vi "Split Host Port.vi"(10 "Address":string) -> (1 "Port":i32, 2 "Hostname":string)   [LabVIEW 2024, in "Sift Client.lvlib" / "Sift Client.lvclass"]
uses:
  Sift Client.lvclass
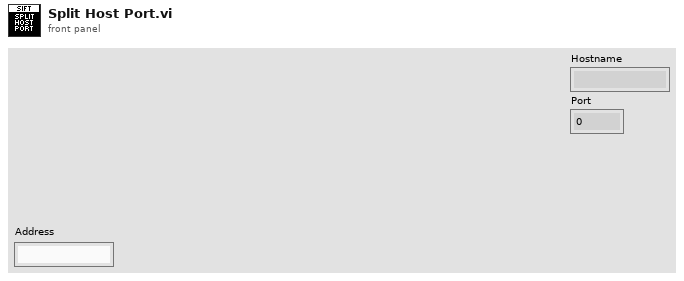
[diagram p1: front panel]
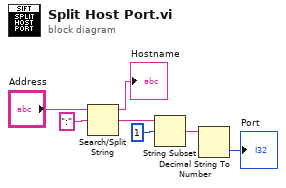
[diagram p0: block diagram]
diagram:
  n1 = Search/Split String(string="Address", search string/char (-)=":") -> (substring before match=→"Hostname":string, match + rest of string=w4:string)  [unwired: 1 in, 1 out]
  n2 = String Subset(string=w4, offset (0)=1) -> (substring=w2:string)  [unwired: 1 in]
  n3 = Decimal String To Number(string=w2) -> (number=→"Port":i32)  [unwired: 2 in, 1 out]
